vi "Channel List Mode Update Cmd.vi"(3 "Current Array":T1=[0, 0, 0, 0, 0], 4 "Pulse Duration":u32[](array[numeric]), 5 "Mode Array":T2) -> (1 "Channel List Mode Init Cmd String":string)   [LabVIEW 2019]
uses:
  Version 2/Data Type Defs/Pulse Mode (array).ctl
  Controls/Stim Current Array.ctl
  Bits Library/Change Bits (U8).vi
  Bits Library/Change Bit (U8).vi
  Bits Library/Bits.lvlib
panel:
  out "Hex bytes":u8[](array[numeric]) format="%02x"
  out "Binary bytes":u8[](array[numeric]) format="%08b"
  out "7-bit current":bool[](array[boolean])
  out "Input Current":bool[](array[boolean])
  out "PW last 7 bits":bool[](array[boolean])
  out "PW first 2 MSB":bool[](array[boolean])
  out "9-bit pulse duration":bool[](array[boolean])
  out "Input pulse duration":bool[](array[boolean])
  out "Byte #4":u8 format="%08b"
  out "Checksum":u8
  out "Byte #3":u8 format="%08b"
  out "Byte #2":u8 format="%08b"
  out "Byte #1":u8 format="%08b"
  # "This VI implements the Channel List Mode Update command found on p.9 of the Hasomed RehaStim Science Mode documentation (https://issuu.com/anatomicalconcepts/docs/sciencemode_software_for_rehastim)"
  # "INPUTS"
  # "DEBUGGING"
  # "OUTPUTS"
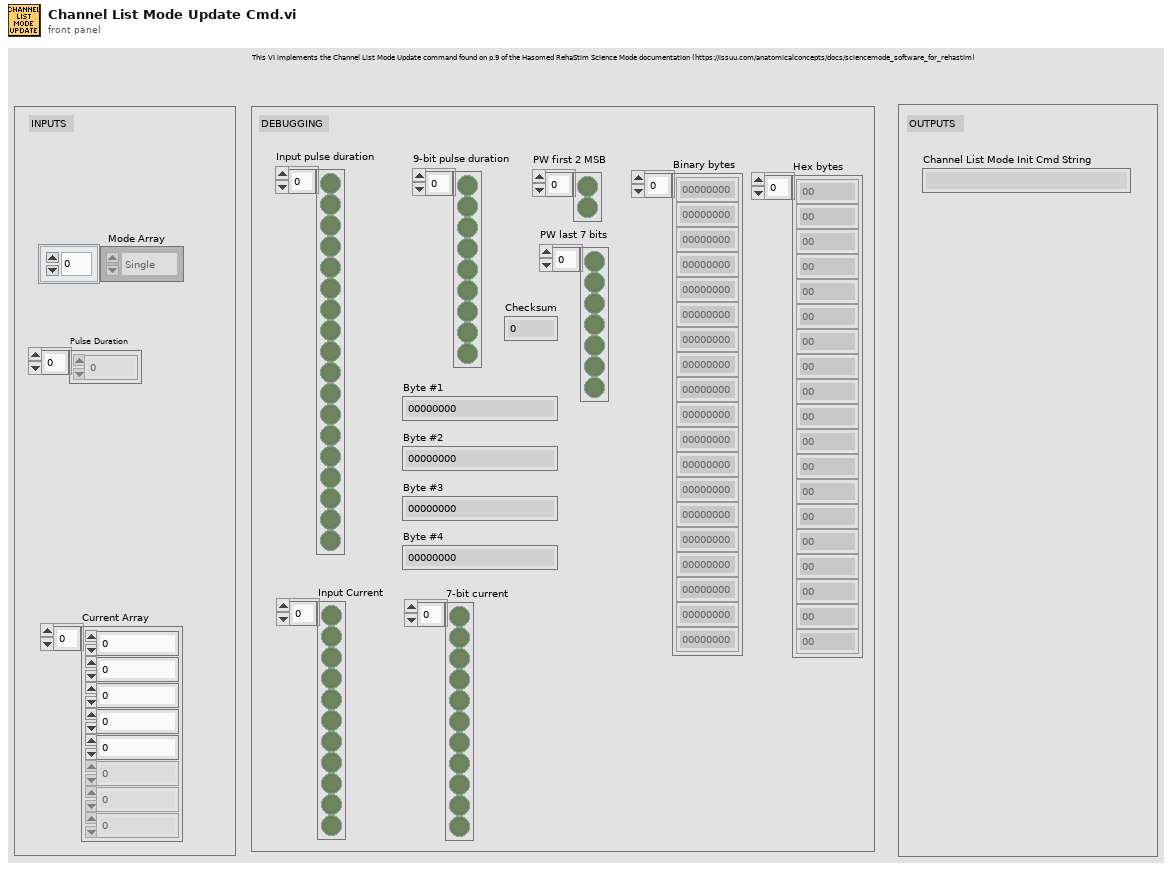
[diagram p1: front panel]
types:
  T1 = typedef "Stim Current Array.ctl" = u8[]
  T2 = typedef "Pulse Mode (array).ctl" = enum16{"Single", "Doublet", "Triplet"}[]
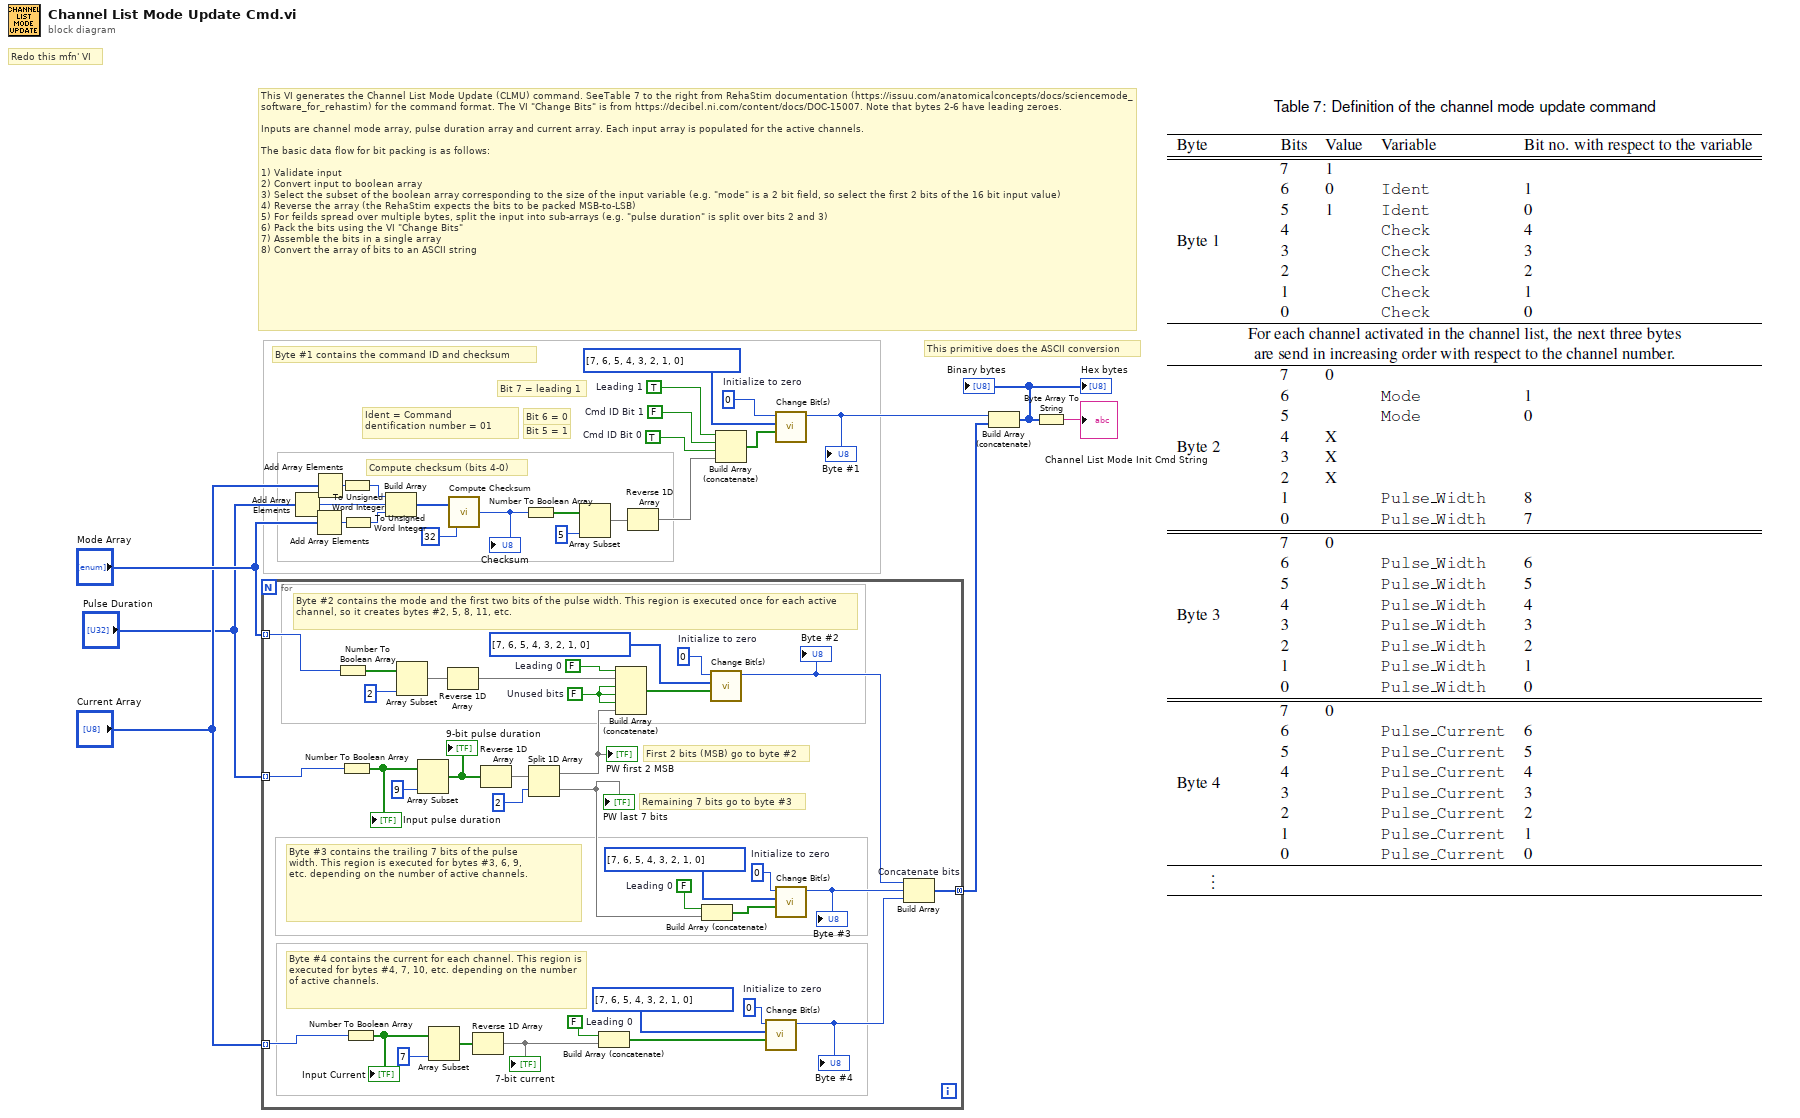
[diagram p0: block diagram]
diagram:
  w21 = TRUE  # Cmd ID Bit 0
  w22 = FALSE  # Cmd ID Bit 1
  w23 = TRUE  # Leading 1
  w25 = u8 0  # Initialize to zero
  # "Redo this mfn' VI"
  # "Compute checksum (bits 4-0)"
  # "Bit 5 = 1"
  # "Bit 6 = 0"
  # "Bit 7 = leading 1"
  # "Byte #1 contains the command ID and checksum"
  # "Ident = Command \ndentification number = 01"
  # "This primitive does the ASCII conversion"
  # "This VI generates the Channel List Mode Update (CLMU) command. SeeTable 7 to the right from RehaStim documentation (https://issuu.com/anatomicalconcepts/docs/sciencemode_software_for_rehastim) for the command format. The VI \"Change Bits\" is from https://decibel.ni.com/content/docs/DOC-15007. Note that bytes 2-6 have leading zeroes.\n\nInputs are channel mode array, pulse duration array and current array. Each input array is populated for the active channels.\n\nThe basic data flow for bit packing is as follows:\n\n1) Validate input\n2) Convert input to boolean array\n3) Select the subset of the boolean array corresponding to the size of the input variable (e.g. \"mode\" is a 2 bit field, so select the first 2 bits of the 16 bit input value)\n4) Reverse the array (the RehaStim expects the bits to be packed MSB-to-LSB)\n5) For feilds spread over multiple bytes, split the input into sub-arrays (e.g. \"pulse duration\" is split over bits 2 and 3)\n6) Pack the bits using the VI \"Change Bits\"\n7) Assemble the bits in a single array\n8) Convert the array of bits to an ASCII string"
  n1 = for {
    tunnel: "Current Array" -> [w28] mode=indexing
    tunnel: "Pulse Duration" -> [w27] mode=indexing
    tunnel: [w29] -> w10 mode=concatenating
    tunnel: "Mode Array" -> [w26] mode=indexing
    w38 = FALSE  # Leading 0
    w40 = u8 0  # Initialize to zero
    w44 = FALSE  # Leading 0
    w46 = u8 0  # Initialize to zero
    w54 = FALSE  # Unused bits
    w53 = FALSE  # Leading 0
    w56 = u8 0  # Initialize to zero
    # "Byte #4 contains the current for each channel. This region is executed for bytes #4, 7, 10, etc. depending on the number of active channels."
    # "Remaining 7 bits go to byte #3"
    # "Byte #3 contains the trailing 7 bits of the pulse\nwidth. This region is executed for bytes #3, 6, 9,\netc. depending on the number of active channels."
    # "First 2 bits (MSB) go to byte #2"
    # "Byte #2 contains the mode and the first two bits of the pulse width. This region is executed once for each active channel, so it creates bytes #2, 5, 8, 11, etc."
    n2 = Number To Boolean Array(number=w26) -> (Boolean array=w58:bool[])
    n3 = Number To Boolean Array(number=w27) -> (Boolean array=w50:bool[])
    "Input pulse duration" <- w50
    n4 = Number To Boolean Array(number=w28) -> (Boolean array=w35:bool[])
    "Input Current" <- w35
    n5 = Array Subset(array=w58, length=2) -> (w57:bool[])  [unwired: 1 in]
    n6 = Array Subset(array=w50, length=9) -> (w51:bool[])  [unwired: 1 in]
    "9-bit pulse duration" <- w51
    n7 = Array Subset(array=w35, length=7) -> (w34:bool[])  [unwired: 1 in]
    n8 = Reverse 1D Array(array=w57) -> (reversed array=w55:bool[])
    n9 = Reverse 1D Array(array=w34) -> (reversed array=w33:bool[])
    "7-bit current" <- w33
    n10 = Reverse 1D Array(array=w51) -> (reversed array=w49:bool[])
    n11 = Split 1D Array(array=w49, index=2 ("length")) -> (first subarray=w47:bool[], second subarray=w43:bool[])
    "PW first 2 MSB" <- w47
    "PW last 7 bits" <- w43
    n12 = Build Array (concatenate)(w38, w33) -> (w37:bool[])
    n13 = Build Array (concatenate)(w53, w55, w54, w54, w54, w47) -> (w41:bool[])
    n14 = Build Array (concatenate)(w44, w43) -> (w42:bool[])
    n15 = call-poly "Change Bit(s).vi"("Values"=w41, "Bits"=u8[] [7, 6, 5, 4, 3, 2, 1, 0], "Number"=w56) -> ("Number Out"=w32:u8)  [unwired: 8 in]
    "Byte #2" <- w32
    n16 = call-poly "Change Bit(s).vi"("Values"=w37, "Bits"=u8[] [7, 6, 5, 4, 3, 2, 1, 0], "Number"=w40) -> ("Number Out"=w30:u8)  [unwired: 8 in]
    "Byte #4" <- w30
    n17 = call-poly "Change Bit(s).vi"("Values"=w42, "Bits"=u8[] [7, 6, 5, 4, 3, 2, 1, 0], "Number"=w46) -> ("Number Out"=w31:u8)  [unwired: 8 in]
    "Byte #3" <- w31
    n18 = Build Array "Concatenate bits"(w32, w31, w30) -> (w29:u8[])
  }
  n19 = Add Array Elements(numeric array="Pulse Duration") -> (sum=w6:u32)
  n20 = Add Array Elements(numeric array="Mode Array") -> (sum=w8:enum16{"Single", "Doublet", "Triplet"})
  n21 = Add Array Elements(numeric array="Current Array") -> (sum=w7:u8)
  n22 = To Unsigned Word Integer(number=w7) -> (unsigned 16bit integer=w3:u16)
  n23 = To Unsigned Word Integer(number=w8) -> (unsigned 16bit integer=w4:u16)
  n24 = Build Array(w3, w6, w4) -> (w12:u32[])
  n25 = call "Compute Checksum.vi"("Divisor"=32, "Array"=w12) -> ("Checksum"=w14:u8)
  "Checksum" <- w14
  n26 = Number To Boolean Array(number=w14) -> (Boolean array=w17:bool[])
  n27 = Array Subset(array=w17, length=5) -> (w16:bool[])  [unwired: 1 in]
  n28 = Reverse 1D Array(array=w16) -> (reversed array=w15:bool[])
  n29 = Build Array (concatenate)(w23, w22, w21, w15) -> (w20:bool[])
  n30 = call-poly "Change Bit(s).vi"("Values"=w20, "Bits"=u8[] [7, 6, 5, 4, 3, 2, 1, 0], "Number"=w25) -> ("Number Out"=w11:u8)  [unwired: 8 in]
  "Byte #1" <- w11
  n31 = Build Array (concatenate)(w11, w10) -> (w9:u8[])
  "Binary bytes" <- w9
  "Hex bytes" <- w9
  n32 = Byte Array To String(unsigned byte array=w9) -> (string=→"Channel List Mode Init Cmd String":string)
